vi "IS Set Standard Headers.vi"(8 "error in (no error)":errorcluster, 10 "Accepted-Version Optional":string="~0", 11 "client handle":T1) -> (0 "error out":errorcluster, 3 "client handle out":T1)   [LabVIEW 2013]
uses:
  <vilib>/httpClient/LabVIEWHTTPClient.lvlib
  <vilib>/httpClient/ClientHandle.ctl
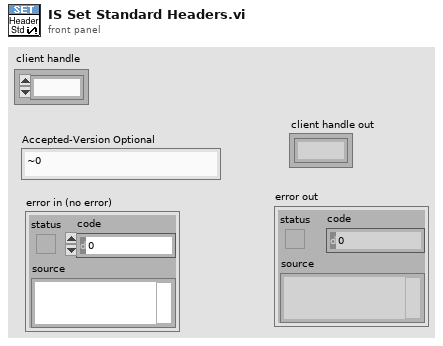
[diagram p1: front panel]
types:
  T1 = typedef "LabVIEWHTTPClient.lvlib/ClientHandle.ctl" = refnum<k1>
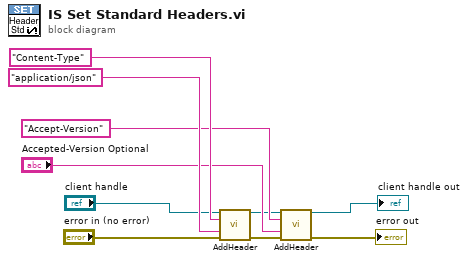
[diagram p0: block diagram]
diagram:
  n1 = call <vilib>:"AddHeader.vi"("client handle"="client handle", "header"="Content-Type", "value"="application/json", "error in (no error)"="error in (no error)") -> ("client handle out"=w4:T1, "error out"=w3:errorcluster)  [unwired: 10 in]
  n2 = call <vilib>:"AddHeader.vi"("client handle"=w4, "header"="Accept-Version", "value"="Accepted-Version Optional", "error in (no error)"=w3) -> ("client handle out"=→"client handle out":T1, "error out"=→"error out":errorcluster)  [unwired: 10 in]
